vi "Move Pixel.vi"(9 "to":T1, 10 "from":T1, 11 "Picture in":refnum<class "Picture.lvclass">) -> (3 "Picture out":refnum<class "Picture.lvclass">)   [LabVIEW 2018]
uses:
  Picture.lvclass
  Coords.ctl
  Picture.lvclass/Picture.ctl
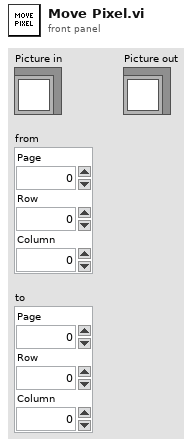
[diagram p1: front panel]
types:
  T1 = typedef "Coords.ctl" = cluster{"Page":i32, "Row":i32, "Column":i32}
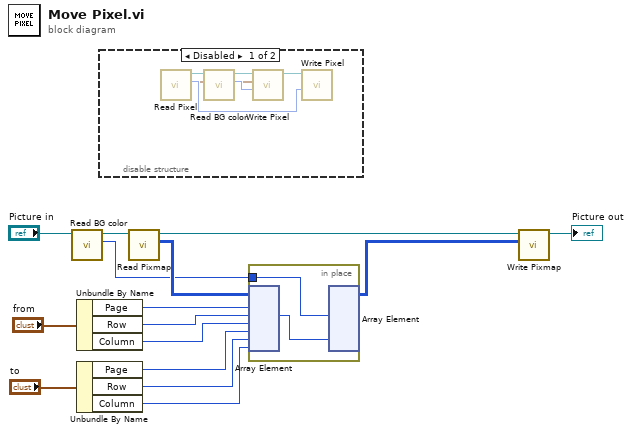
[diagram p0: block diagram]
diagram:
  n1 = call "Read BG color.vi"("Picture in"="Picture in") -> ("BG color"=w6:u32, "Picture out"=w14:refnum<class "Picture.lvclass">)  [unwired: 8 in, 1 out]
  n2 = Unbundle By Name("from") -> ("Page"=w9:i32, "Row"=w8:i32, "Column"=w7:i32)
  n3 = Unbundle By Name("to") -> ("Page"=w4:i32, "Row"=w3:i32, "Column"=w2:i32)
  n4 = disable-structure shown="Disabled" {
    frame Disabled {
      n5 = call "Read Pixel.vi"() -> ("Color"=w22:u32, "Picture out"=w17:refnum<class "Picture.lvclass">, "indices"=w19:T1)  [unwired: 8 in, 1 out]
      n6 = call "Read BG color.vi"("Picture in"=w17) -> ("BG color"=w20:u32, "Picture out"=w18:refnum<class "Picture.lvclass">)  [unwired: 8 in, 1 out]
      n7 = call "Write Pixel.vi"("Color"=w20, "indices"=w19, "Picture in"=w18) -> ("Picture out"=w21:refnum<class "Picture.lvclass">)  [unwired: 7 in, 1 out]
      n8 = call "Write Pixel.vi"("Color"=w22, "Picture in"=w21) -> ("indices"=w16:T1)  [unwired: 7 in, 2 out]
    }
    frame Enabled {
    }
  }
  n9 = call "Read Pixmap.vi"("Picture in"=w14) -> ("3D Pixmap"=w11:u32[][][], "Picture out"=w13:refnum<class "Picture.lvclass">)  [unwired: 8 in, 1 out]
  n10 = in-place {
    in-place-border: w6 -> [w24]
    n11 = in-place-array #1(w11, w9, w8, w7, w4, w3, w2) -> (w23:u32)  [unwired: 1 out]
    n12 = in-place-array #1(w24, w23) -> (w1:u32[][][])  [unwired: 6 out]
  }
  n13 = call "Write Pixmap.vi"("3D Pixmap"=w1, "Picture in"=w13) -> ("Picture out"=→"Picture out":refnum<class "Picture.lvclass">)  [unwired: 8 in, 1 out]
